vi "1_Sin(x)(Training).vi"() -> ()   [LabVIEW 2020]
uses:
  <vilib>/Ngene/Deep Learning Toolkit/Toolkit/NN_Train/Controls/NN_Train_Params.ctl
  <vilib>/Ngene/Deep Learning Toolkit/Toolkit/NN_Train/Controls/NN_Train_Optimizer.ctl
  <vilib>/Ngene/Deep Learning Toolkit/Toolkit/NN_Train/Controls/NN_Train_Data_Sampling.ctl
  <vilib>/Ngene/Deep Learning Toolkit/Toolkit/NN_Train/Controls/NN_LR_Policy_Cfg.ctl
  <vilib>/Ngene/Deep Learning Toolkit/Toolkit/NN_Train/Controls/NN_LR_Policy_Type.ctl
  <vilib>/Ngene/Deep Learning Toolkit/Toolkit/NN_Train/Controls/NN_Train_Session_Data.ctl
  <vilib>/Ngene/Deep Learning Toolkit/Toolkit/NN_Layers/Layers/Input/Controls/NN_Layer_Config(Input1D).ctl
  <vilib>/Ngene/Deep Learning Toolkit/Toolkit/NN_Data/Controls/NN_Data_type.ctl
  <vilib>/Ngene/Deep Learning Toolkit/Toolkit/NN_Network/Controls/NN_Save_Before_Destroy_Options.ctl
  <vilib>/Ngene/Deep Learning Toolkit/Toolkit/NN_Network/Controls/NN_Device.ctl
  <vilib>/Ngene/Deep Learning Toolkit/Toolkit/NN_Layers/Layers/FC/Controls/NN_Layer_Config(FC).ctl
  <vilib>/Ngene/Deep Learning Toolkit/Toolkit/NN_Layers/Layers/BatchNorm/Controls/NN_BN_Params.ctl
  <vilib>/Ngene/Deep Learning Toolkit/Toolkit/NN_Activations/Controls/NN_Activation_Type.ctl
  <vilib>/Ngene/Deep Learning Toolkit/Toolkit/NN_Layers/Controls/NN_Layer_Init_Params.ctl
  <vilib>/Ngene/Deep Learning Toolkit/Toolkit/NN_Layers/Controls/NN_Layer_Weight_Init_Type.ctl
  <vilib>/Ngene/Deep Learning Toolkit/Toolkit/NN_Data/API/DataSet/DataSet_Types/NN_DataSet(In1D_Out1D).ctl
  <vilib>/Ngene/Deep Learning Toolkit/Toolkit/NN_Data/Controls/DataRef_Types/2D/NN_Data_ref(2D_SGL).ctl
  <vilib>/Analysis/1siggen.llb/Ramp Pattern by Samples.vi
  <vilib>/Ngene/Deep Learning Toolkit/Toolkit/NN_Layers/Layers/Input/NN_Layer_Create(Input1D).vi
  <vilib>/Ngene/Deep Learning Toolkit/Toolkit/NN_Layers/Layers/FC/NN_Layer_Create(FC).vi
  <vilib>/Ngene/Deep Learning Toolkit/Toolkit/NN_Train/Loss_Functions/NN_Set_Loss(MSE).vi
  <vilib>/Ngene/Deep Learning Toolkit/Toolkit/NN_Data/subVIs/Get_Data_Vals/2D/NN_Data_Get_ValByRef(2D_SGL).vi
  <vilib>/Ngene/Deep Learning Toolkit/Toolkit/NN_Network/subVIs/NN_Predict/NN_Predict(In1D_Out1D).vi
  <vilib>/Ngene/Deep Learning Toolkit/Toolkit/NN_Train/Eval_Loss/NN_Eval_Test_Error_Loss/NN_Eval(In1D_Out1D).vi
  <vilib>/Ngene/Deep Learning Toolkit/Toolkit/Deep_Learning_Toolkit_by_Ngene.lvlib
  <vilib>/Analysis/NI_AALBase.lvlib
panel:
  out "Loop Time":dbl=0.0014889000000266606 format="%#_4p"
  out "Test Loss":sgl=6.473779e-05
  out "Training Loss":sgl=6.795796e-05
  in  "Stop":bool
  out "Loss Chart":cluster{"Loss":sgl, "Test Loss":sgl}(graph)={"Loss"=6.795796e-05, "Test Loss"=6.473779e-05}
  in  "# of Sine Cycles":dbl=4.0
  out "Sin(x): Predictions vs Ground Truths":sgl[][](graph)
  in  "Eval?":bool
  out "Session Data":T1={"Epochs"=1922.368, "Tot_Iter"=30037, "LR"=1.953125e-05, "LR_iter"=30038}
  in  "LR_Decay_Params":T2={"Policy_Type"=enum."Step", "LR0"=0.01, "k"=200.0, "WarmUp_Policy"=enum."Ramp", "WarmUp_Iter"=100, "WarmUp_Ratio"=10.0} {"WarmUp_Ratio" min=1; "WarmUp_Iter" min=1; "LR0" format="%.7f"}
  in  "NN_Train_Params":T4={"Optimizer"=enum."Adam", "Beta_1"=0.9, "Beta_2"=0.999, "Weight Decay(L1)"=1e-08, "Weight Decay(L2)"=1e-08, "Data_Sampling"=enum."Random"}
  # "Overview: Demonstrates the usage of DeepLTK (Deep Learning Toolkit for LabVIEW) for solving a simple regression problem of modeling sin(x) function.\nRequirements: DeepLTK - Deep Learning Toolkit for LabVIEW (https://www.ngene.co/deep-learning-toolkit-for-labview)\nInstructions:\n1. Run the VI with default configurations.\n2. Observe how the training loss is decreasing.\n3. Periodically press \"Eval?\" button to observe \"Test Loss\" and performance of the model on Test Dataset\n4. Press \"Stop\" when \"Test Loss\" is is not decreasing. ~1500 epochs\nMore Examples:  https://github.com/ngenehub/deepltk_examples"
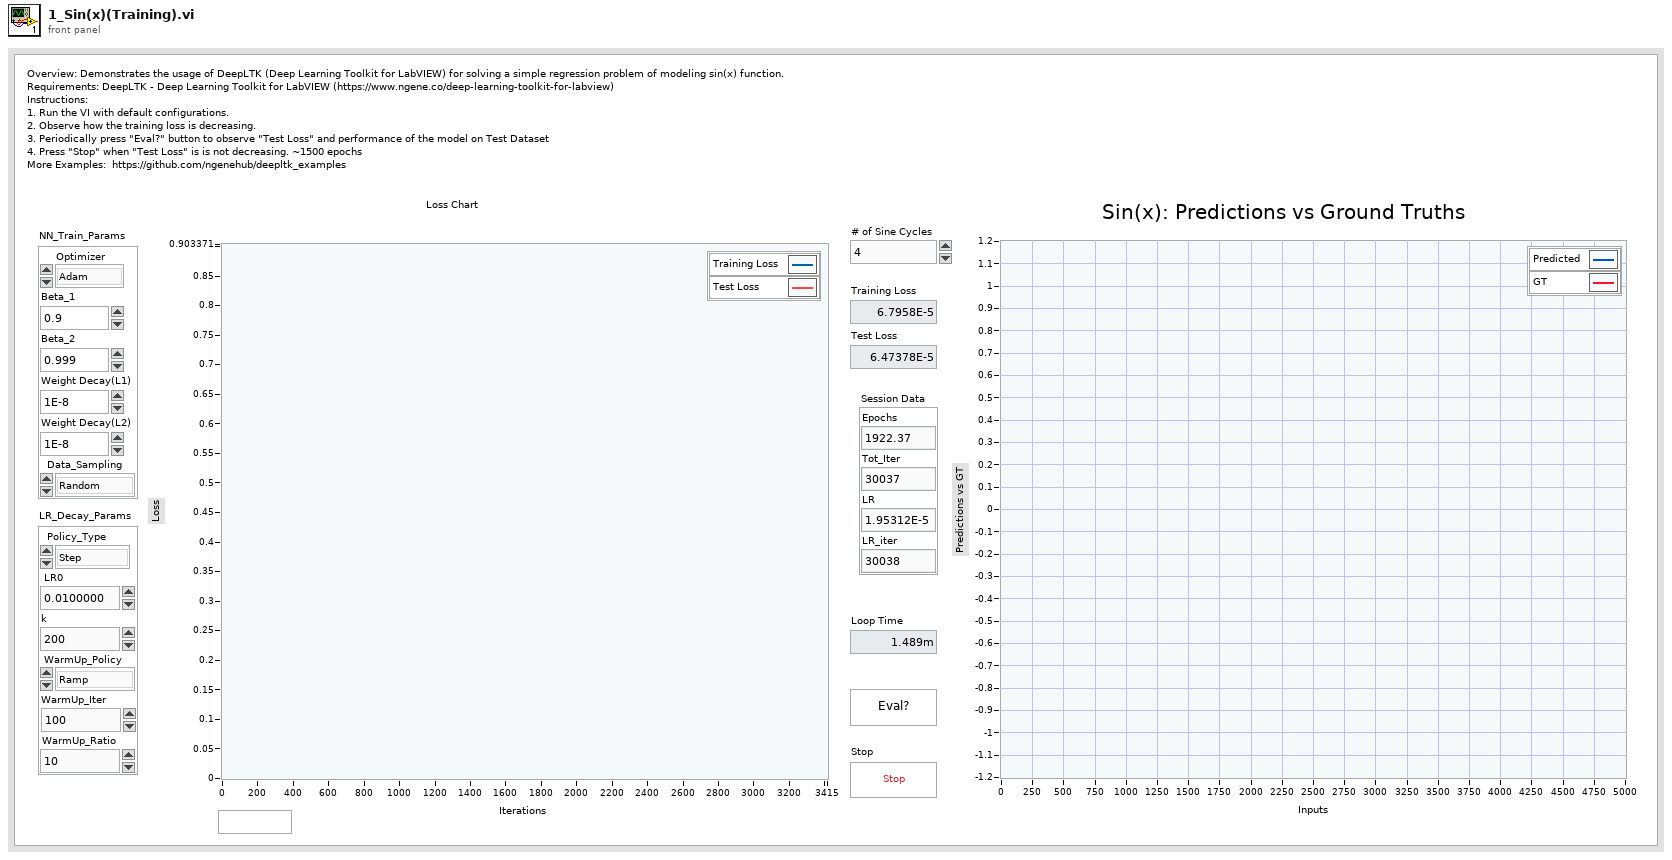
[diagram p1: front panel]
types:
  T1 = typedef "Deep_Learning_Toolkit_by_Ngene.lvlib/NN_Train_Session_Data.ctl" = cluster{"Epochs":sgl, "Tot_Iter":i32, "LR":sgl, "LR_iter":i32}
  T2 = typedef "Deep_Learning_Toolkit_by_Ngene.lvlib/NN_LR_Policy_Cfg.ctl" = cluster{"Policy_Type":T3, "LR0":dbl, "k":sgl, "WarmUp_Policy":enum16{"Step", "Ramp"}, "WarmUp_Iter":i32, "WarmUp_Ratio":sgl}
  T3 = typedef "Deep_Learning_Toolkit_by_Ngene.lvlib/NN_LR_Policy_Type.ctl" = enum16{"Manual", "Step", "Exp", "1/t"}
  T4 = typedef "Deep_Learning_Toolkit_by_Ngene.lvlib/NN_Train_Params.ctl" = cluster{"Optimizer":T5, "Beta_1":sgl, "Beta_2":sgl, "Weight Decay(L1)":sgl, "Weight Decay(L2)":sgl, "Data_Sampling":T6}
  T5 = typedef "Deep_Learning_Toolkit_by_Ngene.lvlib/NN_Train_Optimizer.ctl" = enum16{"SGD", "Adam", "Adagrad", "Adadelta", "RMSProp", "Nesterov"}
  T6 = typedef "Deep_Learning_Toolkit_by_Ngene.lvlib/NN_Train_Data_Sampling.ctl" = enum16{"Random", "Sequential"}
  T7 = typedef "Deep_Learning_Toolkit_by_Ngene.lvlib/NN_Layer_Config(FC).ctl" = cluster{"Name":string, "Size":i32, "BN":bool, "BN_Params":T8, "Activation":T9, "Has Bias?":bool, "Init_Params":T10, "Custom_Params":string}
  T8 = typedef "Deep_Learning_Toolkit_by_Ngene.lvlib/NN_BN_Params.ctl" = cluster{"epsilon":sgl, "momentum":sgl}
  T9 = typedef "Deep_Learning_Toolkit_by_Ngene.lvlib/NN_Activation_Type.ctl" = enum16{"Sigmoid", "ReLU", "LReLU", "ReLU6", "tanh", "Swish", "Mish", "None"}
  T10 = typedef "Deep_Learning_Toolkit_by_Ngene.lvlib/NN_Layer_Init_Params.ctl" = cluster{"Init_Type":T11, "Value":sgl}
  T11 = typedef "Deep_Learning_Toolkit_by_Ngene.lvlib/NN_Layer_Weight_Init_Type.ctl" = enum16{"Const", "Uniform", "Gaussian", "Xavier"}
  T12 = typedef "Deep_Learning_Toolkit_by_Ngene.lvlib/NN_DataSet(In1D_Out1D).ctl" = cluster{"Inputs Ref.":variant, "Outputs Ref.":T13, "Dims_In":i32, "Dataset_Size":i32, "Dims_Out":i32, "Labels":string[], "File Paths":path[]}
  T13 = typedef "Deep_Learning_Toolkit_by_Ngene.lvlib/NN_Data_ref(2D_SGL).ctl" = refnum<data-value>
  T14 = typedef "Deep_Learning_Toolkit_by_Ngene.lvlib/NN_Device.ctl" = enum16{"CPU", "GPU"}
  T15 = typedef "Deep_Learning_Toolkit_by_Ngene.lvlib/NN_Save_Before_Destroy_Options.ctl" = cluster{"CFG?":bool, "Weights?":bool, "Render?":bool}
  T16 = typedef "Deep_Learning_Toolkit_by_Ngene.lvlib/NN_Layer_Config(Input1D).ctl" = cluster{"Name":string, "Size":i32, "Data_Type":T17, "Shift":sgl, "Scale":sgl}
  T17 = typedef "Deep_Learning_Toolkit_by_Ngene.lvlib/NN_Data_type.ctl" = enum16{"I8", "U8", "I16", "U16", "U32 ARGB", "SGL"}
  T18 = typedef "Deep_Learning_Toolkit_by_Ngene.lvlib/NN.ctl" = cluster{"Name":string, "No of Layers":i32, "mBatch":i32, "Layers":T19[], "Dimty":T20, "Dims_In":T21, "Dims_Out":T21, "Working_Dir":path, "Train?":bool, "Train_Params":T4, "LR_Update_Policy":T2, "Session Data":T1, "Ground_truth":T22, "NNg_hdls":T23, "NN_Device":T14, "GPU Id":i32, "Labels":string[], "Receptive Field":T24[], "Loss_Type":T25, "Loss_Cfg_Prms":variant, "NNG_WS":T26}
  T19 = typedef "Deep_Learning_Toolkit_by_Ngene.lvlib/NN_Layer_ref.ctl" = refnum<data-value>
  T20 = typedef "Deep_Learning_Toolkit_by_Ngene.lvlib/NN_In_Out_Dim-ty.ctl" = enum8{"In1D_Out1D", "In3D_Out1D", "In3D_Out3D", "In3D_OutBBox"}
  T21 = typedef "Deep_Learning_Toolkit_by_Ngene.lvlib/NN_Dims(C,H,W).ctl" = cluster{"C":i32, "H":i32, "W":i32}
  T22 = typedef "Deep_Learning_Toolkit_by_Ngene.lvlib/NN_Ground_truth.ctl" = cluster{"Y":variant}
  T23 = typedef "Deep_Learning_Toolkit_by_Ngene.lvlib/nng_cuda_handles.ctl" = cluster{"cudnn":u64, "cublas":u64, "stream":u64, "curand":u64}
  T24 = typedef "Deep_Learning_Toolkit_by_Ngene.lvlib/NN_Dims(V,H).ctl" = cluster{"V":i32, "H":i32}
  T25 = typedef "Deep_Learning_Toolkit_by_Ngene.lvlib/NN_Loss_Type.ctl" = enum16{"None", "MSE", "CrossEntropy", "YOLO_v2", "YOLO_v4"}
  T26 = typedef "Deep_Learning_Toolkit_by_Ngene.lvlib/NNG_WS.ctl" = cluster{"NNG_WS_Mem":T27, "Max_WS_Size":i64}
  T27 = typedef "Deep_Learning_Toolkit_by_Ngene.lvlib/NNg_WS_Mem_DVR.ctl" = refnum<data-value>
  T28 = typedef "Deep_Learning_Toolkit_by_Ngene.lvlib/NN_Eval_Params.ctl" = cluster{"Loss":sgl, "Error":sgl}
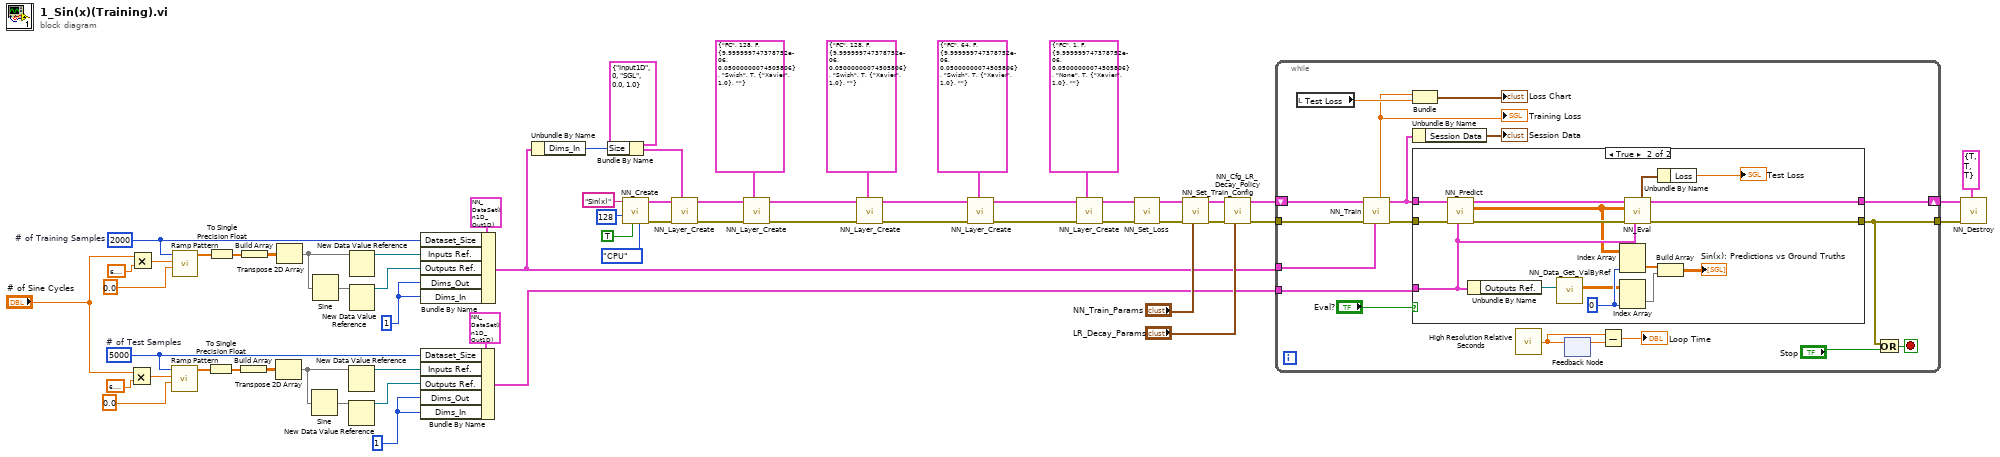
[diagram p0: block diagram]
diagram:
  w7 = 1 ("Dims_Out")
  w9 = 2000  # # of Training Samples
  w21 = 5000  # # of Test Samples
  w22 = 1 ("Dims_Out")
  n1 = Multiply(x="# of Sine Cycles", y=6.283185307179586) -> (x*y=w30:dbl)
  n2 = Multiply(x="# of Sine Cycles", y=6.283185307179586) -> (x*y=w16:dbl)
  n3 = call-poly <vilib>:"Ramp Pattern.vi"("start"=0.0, "end"=w30, "samples"=w21) -> ("Ramp Pattern"=w28:dbl[])  [unwired: 7 in, 1 out]
  n4 = call-poly <vilib>:"Ramp Pattern.vi"("start"=0.0, "end"=w16, "samples"=w9) -> ("Ramp Pattern"=w14:dbl[])  [unwired: 7 in, 1 out]
  n5 = To Single Precision Float(number=w28) -> (single precision float=w29:sgl[])
  n6 = To Single Precision Float(number=w14) -> (single precision float=w15:sgl[])
  n7 = Build Array(w29) -> (w27:sgl[][])
  n8 = Build Array(w15) -> (w13:sgl[][])
  n9 = Transpose 2D Array(2D array=w27) -> (transposed array=w26:sgl[][])
  n10 = Transpose 2D Array(2D array=w13) -> (transposed array=w12:sgl[][])
  n11 = Sine(x=w26) -> (sin(x)=w25:sgl[][])
  n12 = Sine(x=w12) -> (sin(x)=w11:sgl[][])
  n13 = New Data Value Reference(data value=w26) -> (data value reference=w33:refnum<data-value>)  [unwired: 1 in, 1 out]
  n14 = New Data Value Reference(data value=w25) -> (data value reference=w32:refnum<data-value>)  [unwired: 1 in, 1 out]
  n15 = New Data Value Reference(data value=w12) -> (data value reference=w19:refnum<data-value>)  [unwired: 1 in, 1 out]
  n16 = New Data Value Reference(data value=w11) -> (data value reference=w18:refnum<data-value>)  [unwired: 1 in, 1 out]
  n17 = Bundle By Name(cluster=T12 {"Inputs Ref."=variant(refnum<data-value> refnum), "Outputs Ref."=refnum, "Dims_In"=0, "Dataset_Size"=0, "Dims_Out"=0, "Labels"=[], "File Paths"=[]} ("Dataset(In1D_Out1D)"), "Dataset_Size"=w21, "Inputs Ref."=w33, "Outputs Ref."=w32, "Dims_Out"=w22, "Dims_In"=w22) -> (w24:T12)
  n18 = Bundle By Name(cluster=T12 {"Inputs Ref."=variant(refnum<data-value> refnum), "Outputs Ref."=refnum, "Dims_In"=0, "Dataset_Size"=0, "Dims_Out"=0, "Labels"=[], "File Paths"=[]} ("Dataset(In1D_Out1D)"), "Dataset_Size"=w9, "Inputs Ref."=w19, "Outputs Ref."=w18, "Dims_Out"=w7, "Dims_In"=w7) -> (w8:T12)
  n19 = Unbundle By Name(w8) -> ("Dims_In"=w39:i32)
  n20 = Bundle By Name(cluster=T16 {"Name"="Input1D", "Size"=0, "Data_Type"=enum."SGL", "Shift"=0.0, "Scale"=1.0} ("Input1D_Cfg"), "Size"=w39) -> (w55:T16)
  n21 = call <vilib>:"NN_Create.vi"("NN_Device"=NN_Device."CPU", "Train? (false)"=TRUE, "mBatch (1)"=128, "Name"="Sin(x)") -> ("error out"=w60:errorcluster, "NN out"=w61:T18)  [unwired: 6 in]
  n22 = call-poly <vilib>:"NN_Layer_Create.vi"("Input1D_Cfg"=w55, "error in (no error)"=w60, "NN in"=w61) -> ("error out"=w63:errorcluster, "NN out"=w62:T18)  [unwired: 6 in, 1 out]
  n23 = call-poly <vilib>:"NN_Layer_Create.vi"("FC_Cfg"=T7 {"Name"="FC", "Size"=128, "BN"=FALSE, "BN_Params"={"epsilon"=1e-05, "momentum"=0.05}, "Activation"=enum."Swish", "Has Bias?"=TRUE, "Init_Params"={"Init_Type"=enum."Xavier", "Value"=1.0}, "Custom_Params"=""}, "error in (no error)"=w63, "NN in"=w62) -> ("error out"=w36:errorcluster, "NN out"=w37:T18)  [unwired: 6 in, 1 out]
  n24 = call-poly <vilib>:"NN_Layer_Create.vi"("FC_Cfg"=T7 {"Name"="FC", "Size"=128, "BN"=FALSE, "BN_Params"={"epsilon"=1e-05, "momentum"=0.05}, "Activation"=enum."Swish", "Has Bias?"=TRUE, "Init_Params"={"Init_Type"=enum."Xavier", "Value"=1.0}, "Custom_Params"=""}, "error in (no error)"=w36, "NN in"=w37) -> ("error out"=w3:errorcluster, "NN out"=w4:T18)  [unwired: 6 in, 1 out]
  n25 = call-poly <vilib>:"NN_Layer_Create.vi"("FC_Cfg"=T7 {"Name"="FC", "Size"=64, "BN"=FALSE, "BN_Params"={"epsilon"=1e-05, "momentum"=0.05}, "Activation"=enum."Swish", "Has Bias?"=TRUE, "Init_Params"={"Init_Type"=enum."Xavier", "Value"=1.0}, "Custom_Params"=""}, "error in (no error)"=w3, "NN in"=w4) -> ("error out"=w1:errorcluster, "NN out"=w2:T18)  [unwired: 6 in, 1 out]
  n26 = call-poly <vilib>:"NN_Layer_Create.vi"("FC_Cfg"=T7 {"Name"="FC", "Size"=1, "BN"=FALSE, "BN_Params"={"epsilon"=1e-05, "momentum"=0.05}, "Activation"=enum."None", "Has Bias?"=TRUE, "Init_Params"={"Init_Type"=enum."Xavier", "Value"=1.0}, "Custom_Params"=""}, "error in (no error)"=w1, "NN in"=w2) -> ("error out"=w41:errorcluster, "NN out"=w40:T18)  [unwired: 6 in, 1 out]
  n27 = call-poly <vilib>:"NN_Set_Loss.vi"("error in (no error)"=w41, "NN in"=w40) -> ("error out"=w42:errorcluster, "NN out"=w43:T18)  [unwired: 8 in]
  n28 = call <vilib>:"NN_Set_Train_Config.vi"("NN_Train_Params"="NN_Train_Params", "error in (no error)"=w42, "NN in"=w43) -> ("error out"=w48:errorcluster, "NN out"=w53:T18)  [unwired: 7 in]
  n29 = call <vilib>:"NN_Cfg_LR_Decay_Policy.vi"("LR_Decay_Params"="LR_Decay_Params", "error in (no error)"=w48, "NN in"=w53) -> ("error out"=w47:errorcluster, "NN out"=w49:T18)  [unwired: 7 in]
  n30 = while {
    tunnel: w47 -> [w80]
    tunnel: w8 -> [w65]
    shift-right: [w76] -> w51
    shift-left: w49 -> [w81]
    tunnel: [w72] -> w50
    tunnel: w24 -> [w64]
    stop <- w79 stop-if-true
    n31 = local read "Test Loss"() -> (w73:sgl)
    n32 = call <vilib>:"NN_Train.vi"("Train Dataset"=w65, "error in (no error)"=w80, "NN in"=w81) -> ("error out"=w75:errorcluster, "NN out"=w78:T18, "Loss"=w66:sgl)  [unwired: 3 in, 3 out]
    "Training Loss" <- w66
    n33 = Bundle("Loss"=w66, "Test Loss"=w73) -> (→"Loss Chart":cluster{"Loss":sgl, "Test Loss":sgl})  [unwired: 1 in]
    n34 = Unbundle By Name(w78) -> ("Session Data"=→"Session Data":T1)
    n35 = case shown="True" "Eval?" {
      tunnel: w78 -> [w83 w95]
      tunnel: [w83 w99] -> w76
      tunnel: w75 -> [w82 w94]
      tunnel: [w82 w98] -> w72
      tunnel: w64 -> [_ w93]
      frame False {
      }
      frame True {
        w90 = 0 ("disabled index (col)")
        n36 = call-poly <vilib>:"NN_Predict.vi"("Dataset"=w93, "error in (no error)"=w94, "NN in"=w95) -> ("error out"=w96:errorcluster, "Predictions"=w91:sgl[][], "NN out"=w97:T18)  [unwired: 6 in]
        n37 = Unbundle By Name(w93) -> ("Outputs Ref."=w92:T13)
        n38 = call-poly <vilib>:"NN_Data_Get_ValByRef.vi"("DVR(2D_SGL)"=w92) -> ("Value(2D_SGL)"=w87:sgl[][])  [unwired: 7 in, 1 out]
        n39 = Index Array(array=w91, index (col)=w90) -> (element=w86:sgl[])  [unwired: 1 in]
        n40 = Index Array(array=w87, index (col)=w90) -> (element=w89:sgl[])  [unwired: 1 in]
        n41 = call-poly <vilib>:"NN_Eval.vi"("Dataset"=w93, "error in (no error)"=w96, "Predictions"=w91, "NN in"=w97) -> ("error out"=w98:errorcluster, "NN out"=w99:T18, "NN_Eval_Params"=w85:T28)  [unwired: 4 in, 1 out]
        n42 = Unbundle By Name(w85) -> ("Loss"=→"Test Loss":sgl)
        n43 = Build Array(w86, w89) -> (→"Sin(x): Predictions vs Ground Truths":sgl[][])
      }
    }
    n44 = call <vilib>:"High Resolution Relative Seconds.vi"() -> ("relative seconds"=w71:dbl)
    n45 = feedback-in #1(w71) -> ()
    n46 = feedback #1() -> (w70:dbl)  [unwired: 1 in]
    n47 = Subtract(x=w71, y=w70) -> (x-y=→"Loop Time":dbl)
    n48 = Or(x=w72, y="Stop") -> (x .or. y?=w79:bool)
  }
  n49 = call <vilib>:"NN_Destroy.vi"("Save (T, T, T)"=T15 {"CFG?"=TRUE, "Weights?"=TRUE, "Render?"=TRUE}, "error in (no error)"=w50, "NN in"=w51) -> ()  [unwired: 7 in, 2 out]
